vi "DCPower_InstrumentArrayCheck.vi"(8 "error in (no error)":errorcluster, 10 "DCPowerInformationClusterArray_Input":T1[](array[typedef]), 11 "IVI Refnum in":refnum<k15>) -> (0 "error out":errorcluster, 1 "IVI Ref index":i32, 2 "IVI Ref Present?":bool, 3 "IVI Refnum out":refnum<k15>)   [LabVIEW 2019]
uses:
  Controls/DCPowerBlock_byInstrument_Control.ctl
panel:
  in  "DCPowerInformationClusterArray_Input":T2(array[cluster])
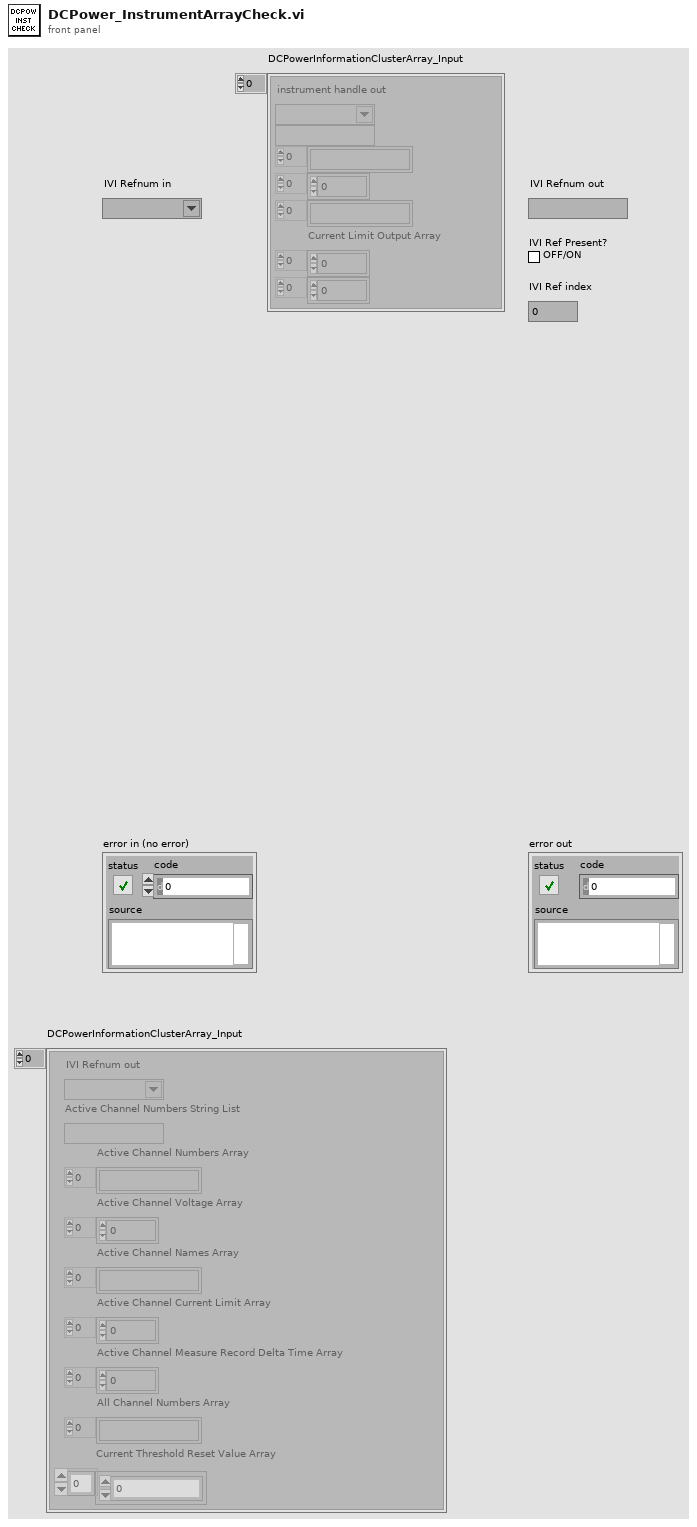
[diagram p1: front panel]
types:
  T1 = typedef "DCPowerBlock_byInstrument_Control.ctl" = cluster{"IVI Refnum out":refnum<k15>, "Active Channel Numbers String List":string, "Active Channel Numbers Array":string[], "Active Channel Voltage Array":dbl[], "Active Channel Names Array":string[], "Active Channel Current Limit Array":dbl[], "Active Channel Measure Record Delta Time Array":dbl[], "All Channel Numbers Array":string[], "Current Threshold Reset Value Array":dbl[]}
  T2 = cluster{"instrument handle out":refnum<k15>, string, string[], dbl[], string[], "Current Limit Output Array":dbl[], dbl[]}[]
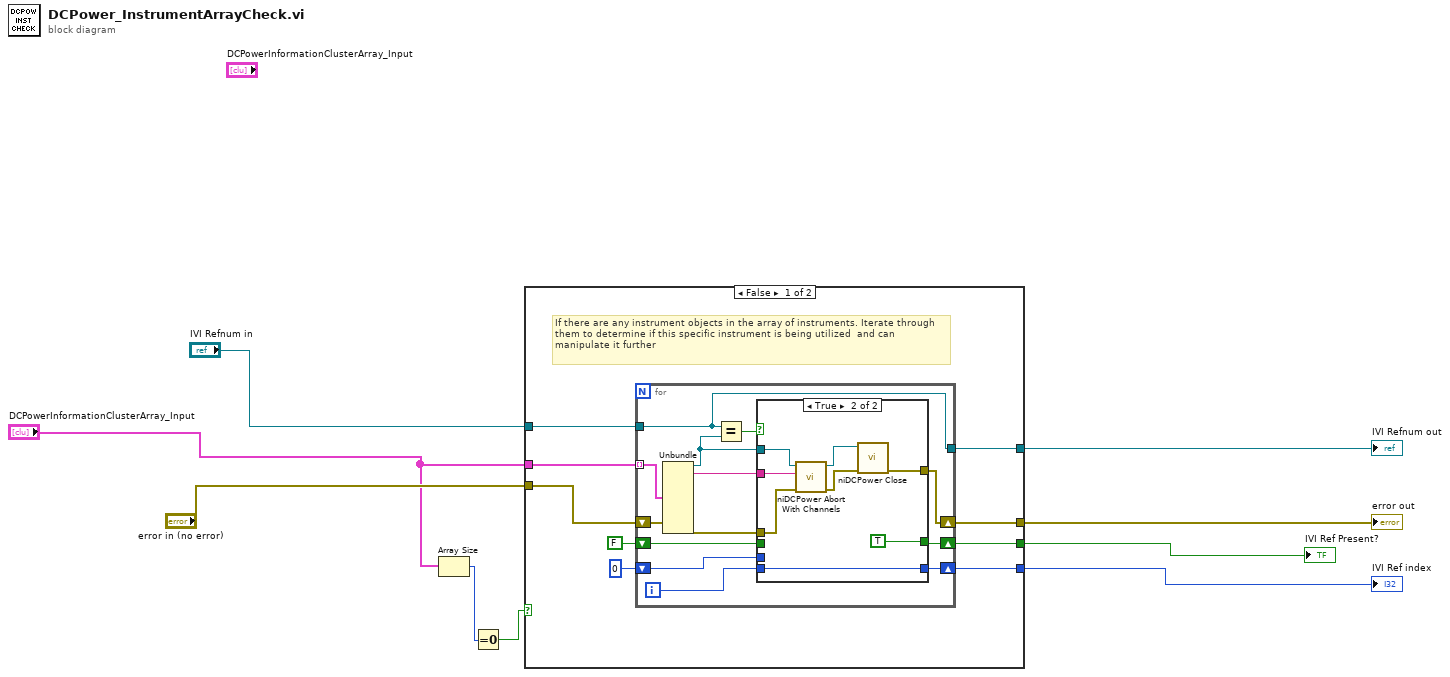
[diagram p0: block diagram]
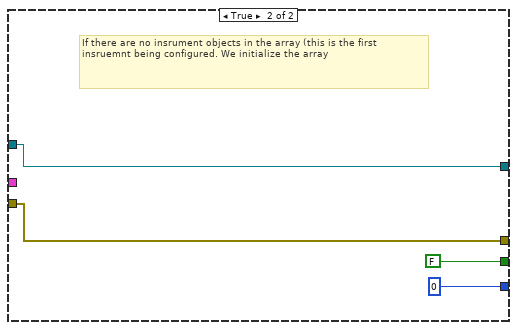
[diagram p3: hidden frame]
diagram:
  n1 = Array Size(array="DCPowerInformationClusterArray_Input") -> (size(s)=w3:i32)
  n2 = Equal To 0?(x=w3) -> (x = 0?=w2:bool)
  n3 = case shown="False" w2 {
    tunnel: [w18 w45] -> w9
    tunnel: [w17 0] -> w8
    tunnel: [w16 FALSE] -> w7
    tunnel: [w15 w44] -> w6
    tunnel: "error in (no error)" -> [w12 w44]
    tunnel: "IVI Refnum in" -> [w11 w45]
    tunnel: "DCPowerInformationClusterArray_Input" -> [w10 _]
    frame False {
      # "If there are any instrument objects in the array of instruments. Iterate through them to determine if this specific instrument is being utilized  and can manipulate it further"
      n4 = for {
        tunnel: w10 -> [w30] mode=indexing
        tunnel: w11 -> [w20]
        shift-right: [w26] -> w17
        shift-left: 0 -> [w24]
        shift-right: [w21] -> w16
        shift-left: FALSE -> [w22]
        shift-right: [w23] -> w15
        shift-left: w12 -> [w27]
        tunnel: [w20] -> w18
        i -> [w25]
        n5 = Unbundle(w30) -> ("IVI Refnum out"=w28:refnum<k15>, "Active Channel Numbers String List"=w19:string)  [unwired: 7 out]
        n6 = Equal?(x=w20, y=w28) -> (x = y?=w29:bool)
        n7 = case shown="True" w29 {
          tunnel: w28 -> [_ w38]
          tunnel: w27 -> [w33 w34]
          tunnel: [w31 w41] -> w26
          tunnel: w25 -> [_ w41]
          tunnel: w24 -> [w31 _]
          tunnel: [w32 TRUE] -> w21
          tunnel: [w33 w39] -> w23
          tunnel: w22 -> [w32 _]
          tunnel: w19 -> [_ w35]
          frame False {
          }
          frame True {
            n8 = call <instrlib>:"niDCPower Abort With Channels.vi"("error in (no error)"=w34, "channel name"=w35, "instrument handle"=w38) -> ("error out"=w37:errorcluster, "instrument handle out"=w36:refnum<k15>)  [unwired: 7 in]
            n9 = call <instrlib>:"niDCPower Close.vi"("error in (no error)"=w37, "instrument handle"=w36) -> ("error out"=w39:errorcluster)  [unwired: 9 in]
          }
        }
      }
    }
    frame True {
      # "If there are no insrument objects in the array (this is the first insruemnt being configured. We initialize the array"
    }
  }
  "IVI Refnum out" <- w9
  "IVI Ref index" <- w8
  "IVI Ref Present?" <- w7
  "error out" <- w6
